vi "Gamma Random.vi"(6 "seed":i32=-1, 7 "reset":bool, 9 "c":dbl=1.0, 10 "b":dbl=1.0, 11 "samples":i32=128) -> (0 "error":i32, 3 "gamma random numbers":dbl[](array[numeric]))   [LabVIEW 2020, in "NI_Gmath.lvlib"]
doc: "Generates random values from a variate X, where X describes the selected distribution type. You must manually select the polymorphic instance to use."
uses:
  <vilib>/gmath/NI_Gmath.lvlib
panel:
  # "Gamma Random"
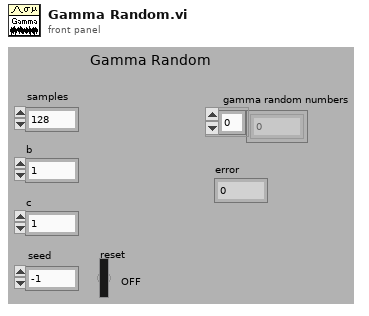
[diagram p1: front panel]
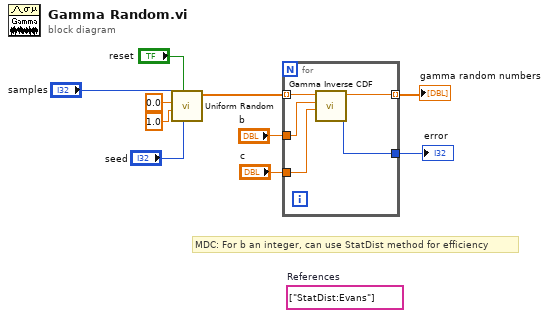
[diagram p0: block diagram]
diagram:
  (unwired) string[] ["StatDist:Evans"]  # References
  # "MDC: For b an integer, can use StatDist method for efficiency"
  n1 = call <vilib>:"Uniform Random.vi"("seed"="seed", "reset"="reset", "xmax"=1.0, "xmin"=0.0, "samples"="samples") -> ("uniform random data"=w3:dbl[])  [unwired: 5 in, 1 out]
  n2 = for {
    tunnel: "b" -> [w15]
    tunnel: "c" -> [w14]
    tunnel: [w13] -> w8 mode=indexing
    tunnel: [w12] -> w7
    tunnel: w3 -> [w11] mode=indexing
    n3 = call <vilib>:"Gamma Inverse CDF.vi"("c"=w14, "b"=w15, "cdf(x)"=w11) -> ("error"=w12:i32, "x"=w13:dbl)  [unwired: 7 in]
  }
  "error" <- w7
  "gamma random numbers" <- w8
